vi "Initialize.vi"(8 "error in (no error)":errorcluster, 9 "type":string=".csv", 10 "Path":path, 11 "Saving OO in":refnum<class "Saving OO.lvclass">) -> (0 "error out":errorcluster, 3 "Saving OO out":refnum<class "Saving OO.lvclass">)   [LabVIEW 2020, in "Saving OO.lvclass"]
uses:
  Saving OO.lvclass
  Saving OO.lvclass/Saving OO.ctl
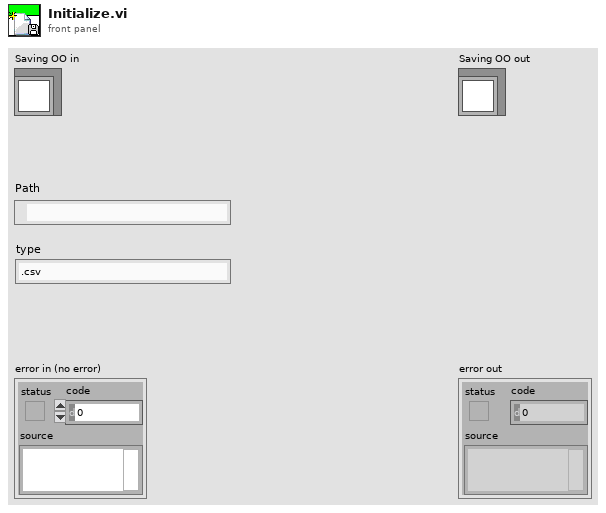
[diagram p1: front panel]
types:
  T1 = enum16{"open", "replace", "create", "open or create", "replace or create", "replace or create with confirmation"}
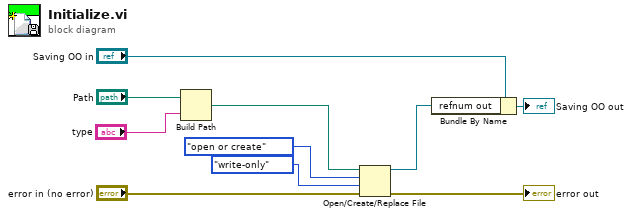
[diagram p0: block diagram]
diagram:
  n1 = Build Path(base path="Path", name or relative path="type") -> (appended path=w4:path)
  n2 = Open/Create/Replace File(file path (use dialog)=w4, error in="error in (no error)", operation (0:open)=T1."open or create", access (0:read/write)=enum16{"read/write", "read-only", "write-only"}."write-only") -> (refnum out=w1:refnum<file>, error out=→"error out":errorcluster)  [unwired: 2 in, 1 out]
  n3 = Bundle By Name(cluster="Saving OO in", "refnum out"=w1) -> (→"Saving OO out":refnum<class "Saving OO.lvclass">)
